vi "Get Class Info.vi"(8 "error in (no error)":errorcluster, 11 "Base Class Name":string) -> (0 "error out":errorcluster, 1 "Success?":bool, 2 "Is Interface?":bool, 3 "Class Info":T1)   [LabVIEW 2020, in "ClassLoader.lvlib"]
doc: "Return info about the given class.\nNote that this VI does not use the cache to store data only to find the correct config file to read from!\n\nThis VI does not automatically load data. Front-load before calling this VI!"
uses:
  ClassLoader.lvlib
  Sub/Ctl/Ctl_Class Info.ctl
  Sub/Cache/Cache_Info Global.vi
  <vilib>/Utility/config.llb/NI_LVConfig.lvlib
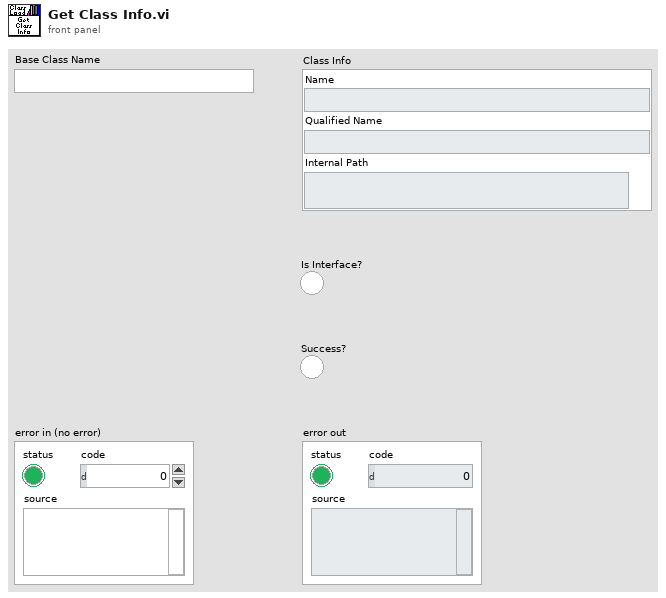
[diagram p1: front panel]
types:
  T1 = typedef "ClassLoader.lvlib/Ctl_Class Info.ctl" = cluster{"Name":string, "Qualified Name":string, "Internal Path":string}
  T2 = typedef "NI_LVConfig.lvlib/Config Data RefNum.ctl" = refnum<k1>
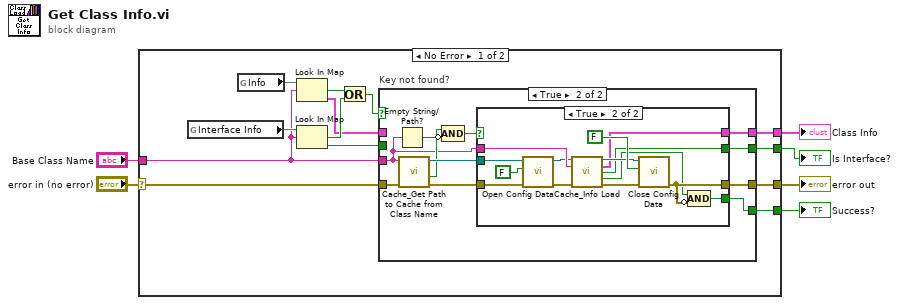
[diagram p0: block diagram]
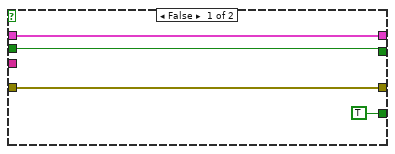
[diagram p2: hidden frame]
diagram:
  n1 = case shown="No Error" "error in (no error)" {
    selector: "error in (no error)" -> [w17 w50]
    tunnel: "Base Class Name" -> [w12 _]
    tunnel: [w18 w50] -> w4
    tunnel: [w19 _] -> w3
    tunnel: [w16 _] -> w2
    tunnel: [w15 _] -> w1
    frame No Error {
      n2 = global read "Cache_Info Global.vi" "Interface Info"() -> (w13:map{string, bool})
      n3 = global read "Cache_Info Global.vi" "Info"() -> (w14:map{string, T1})
      n4 = Look In Map(map=w14, key=w12) -> (key not found?=w10:bool, value=w8:T1)  [unwired: 1 in]
      n5 = Look In Map(map=w13, key=w12) -> (key not found?=w11:bool, value=w7:bool)  [unwired: 1 in]
      n6 = Or(x=w10, y=w11) -> (x .or. y?=w9:bool)
      n7 = case "Key not found?" shown="True" w9 {
        tunnel: [TRUE w31] -> w19
        tunnel: [w21 w30] -> w18
        tunnel: w17 -> [w21 w29]
        tunnel: [w23 w28] -> w16
        tunnel: [w22 w27] -> w15
        tunnel: w12 -> [_ w24]
        tunnel: w8 -> [w23 _]
        tunnel: w7 -> [w22 _]
        frame False {
        }
        frame True {
          n8 = Empty String/Path?(string/path=w24) -> (empty?=w25:bool)
          n9 = call "Cache_Get Path to Cache from Class Name.vi"("error in (no error)"=w29, "Class Name"=w24) -> ("error out"=w32:errorcluster, "Success?"=w33:bool, "Cache Path"=w34:path)  [unwired: 7 in]
          n10 = Compound Arithmetic op=AND(w33, invert w25) -> (w26:bool)
          n11 = case shown="True" w26 {
            tunnel: w34 -> [_ w47]
            tunnel: w24 -> [_ w42]
            tunnel: w32 -> [w35 w46]
            tunnel: [w35 w45] -> w30
            tunnel: [_ w44] -> w31
            tunnel: [_ w39] -> w28
            tunnel: [_ w38] -> w27
            frame False {
            }
            frame True {
              n12 = call <vilib>:"Open Config Data.vi"("error in (no error)"=w46, "create file if necessary (T)"=FALSE, "configuration file path"=w47) -> ("error out"=w36:errorcluster, "refnum"=w37:T2)  [unwired: 6 in, 1 out]
              n13 = call "Cache_Info Load.vi"("Refnum in"=w37, "Class Name"=w42, "error in (no error)"=w36) -> ("Refnum out"=w43:T2, "Class Info"=w39:T1, "Is Interface"=w38:bool, "Success?"=w40:bool, "error out"=w41:errorcluster)  [unwired: 8 in]
              n14 = call <vilib>:"Close Config Data.vi"("error in (no error)"=w41, "write file if changed (T)"=FALSE, "refnum"=w43) -> ("error out"=w45:errorcluster)  [unwired: 7 in, 1 out]
              n15 = Compound Arithmetic op=AND(w40, invert w45) -> (w44:bool)
            }
          }
        }
      }
    }
    frame Error {
    }
  }
  "error out" <- w4
  "Success?" <- w3
  "Class Info" <- w2
  "Is Interface?" <- w1
